vi "Do.vi"(8 "error in (no error)":errorcluster, 10 "Actor in":refnum<class "Actor.lvclass">, 11 "AcquisitionDone Msg":refnum<class "AcquisitionDone Msg.lvclass">) -> (0 "error out":errorcluster, 2 "Actor out":refnum<class "Actor.lvclass">)   [LabVIEW 2023, in "AcquisitionDone Msg.lvclass"]
doc: "This VI delivers the message to the actor by calling the appropriate method(s) on the actor."
uses:
  AcquisitionDone Msg.lvclass
  AcquisitionDone Msg.lvclass/AcquisitionDone Msg.ctl
  fa1874af-2736-4e5f-ab62-8f41ced98009.vi
  Top_Controllers/TopControllerInterface/TopControllerInterface.lvclass
  <vilib>/ActorFramework/Actor/Actor.lvclass
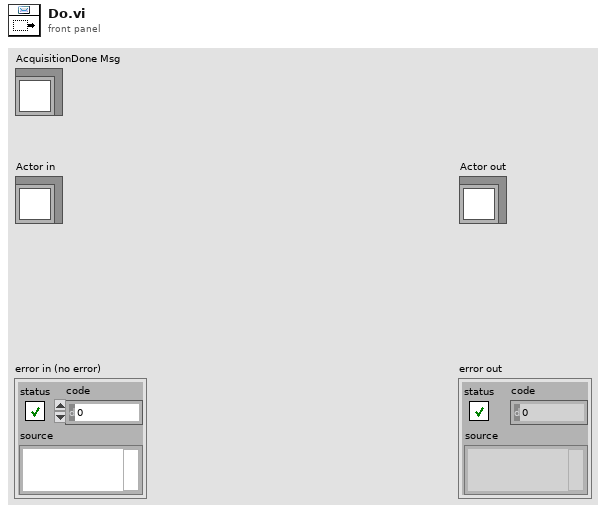
[diagram p1: front panel]
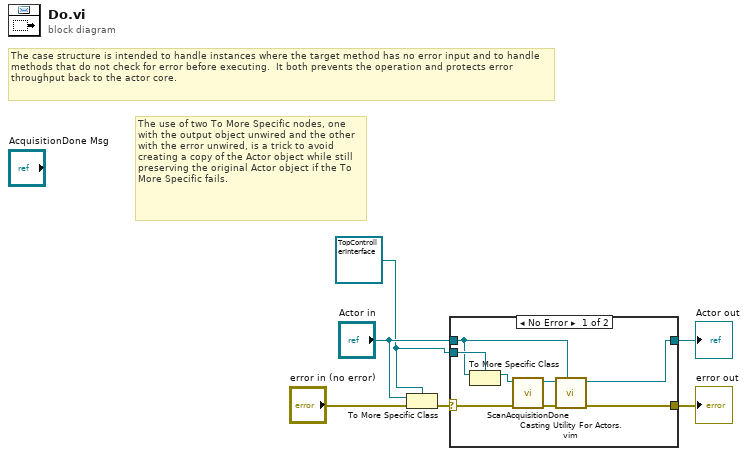
[diagram p0: block diagram]
diagram:
  w1 = refnum<class "TopControllerInterface.lvclass"> refnum ("ControllerComm.lvlib:TopControllerInterface.lvclass")
  # "The use of two To More Specific nodes, one with the output object unwired and the other with the error unwired, is a trick to avoid creating a copy of the Actor object while still preserving the original Actor object if the To More Specific fails."
  # "The case structure is intended to handle instances where the target method has no error input and to handle methods that do not check for error before executing.  It both prevents the operation and protects error throughput back to the actor core."
  n1 = To More Specific Class(target class=w1, reference="Actor in", error in="error in (no error)") -> (error out=w2:errorcluster)  [unwired: 1 out]
  n2 = case shown="No Error" w2 {
    selector: w2 -> [w9 w16]
    tunnel: [w11 w16] -> w6
    tunnel: [w12 w15] -> w5
    tunnel: "Actor in" -> [w13 w15]
    tunnel: w1 -> [w14 _]
    frame No Error {
      n3 = To More Specific Class(target class=w14, reference=w13) -> (specific class reference=w10:refnum<class "TopControllerInterface.lvclass">)  [unwired: 1 in, 1 out]
      n4 = call-dynamic "ScanAcquisitionDone.vi"("error in (no error)"=w9, "ControllerComm.lvlib:TopControllerInterface.lvclass"=w10) -> ("error out"=w7:errorcluster, "ControllerComm.lvlib:TopControllerInterface.lvclass"=w8:refnum<class "TopControllerInterface.lvclass">)  [unwired: 8 in]
      n5 = call "Casting Utility For Actors.vim"("type"=w13, "error in (no error)"=w7, "Actor in"=w8) -> ("error out"=w11:errorcluster, "Actor out"=w12:refnum<class "Actor.lvclass">)  [unwired: 7 in]
    }
    frame Error {
      # "If type check fails, pass the original object out again."
    }
  }
  "error out" <- w6
  "Actor out" <- w5
